vi "PWM.vi"(8 "milliseconds to wait 2":u32=100, 9 "Period (sec) 2":dbl=3.0, 10 "Duty Cycle 2":dbl format="%#_13g", 11 "Starting tic count":u32) -> (1 "Elapsed time (sec) 2":dbl format="%#.3f", 2 "Pwm output 2":dbl)   [LabVIEW 2013]
doc: "Use this template to build a standard state machine design pattern. Each state executes code and determines which state to transition to. Contrast this design pattern with the User Interface Event Handler pattern, in which code executes in response to user actions. Contrast this design pattern also with the Queued Message Handler pattern, in which each message handling code can queue zero or more new messages."
panel:
  out "Elapsed Time":u32
  out "starting tic count or new tic":u32
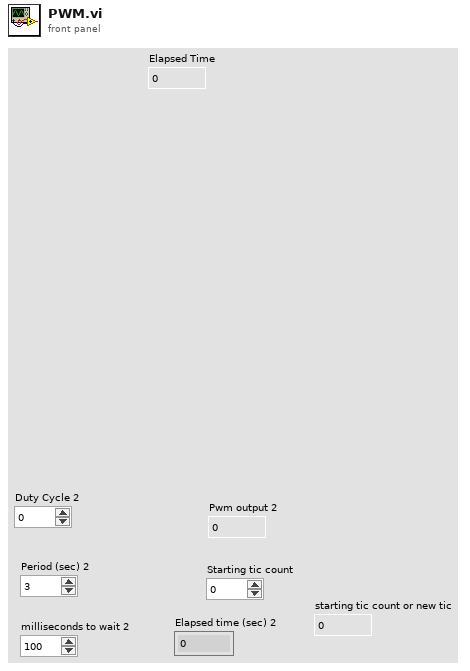
[diagram p1: front panel]
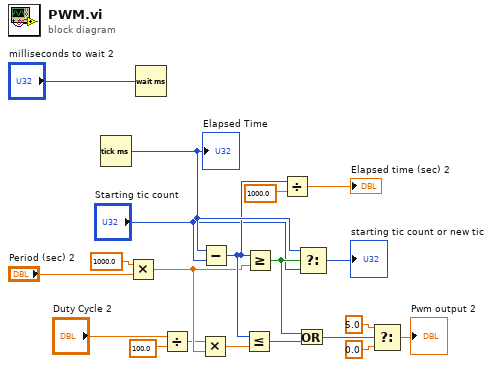
[diagram p0: block diagram]
diagram:
  n1 = Tick Count (ms)() -> (millisecond timer value=w15:u32)
  "Elapsed Time" <- w15
  n2 = Multiply(x=1000.0, y="Period (sec) 2") -> (x*y=w11:dbl)
  n3 = Wait (ms)(milliseconds to wait="milliseconds to wait 2") -> ()  [unwired: 1 out]
  n4 = Divide(x="Duty Cycle 2", y=100.0) -> (x/y=w2:dbl)
  n5 = Multiply(x=w2, y=w11) -> (x*y=w10:dbl)
  n6 = Subtract(x=w15, y="Starting tic count") -> (x-y=w12:u32)
  n7 = Less Or Equal?(x=w12, y=w10) -> (x <= y?=w8:bool)
  n8 = Greater Or Equal?(x=w12, y=w11) -> (x >= y?=w7:bool)
  n9 = Divide(x=w12, y=1000.0) -> (x/y=→"Elapsed time (sec) 2":dbl)
  n10 = Or(x=w7, y=w8) -> (x .or. y?=w9:bool)
  n11 = Select(t=w15, s=w7, f="Starting tic count") -> (s? t:f=→"starting tic count or new tic":u32)
  n12 = Select(t=5.0, s=w9, f=0.0) -> (s? t:f=→"Pwm output 2":dbl)
